vi "process.vi"(8 "error in":errorcluster, 9 "result allocation":T1, 10 "parameters":T1, 11 "module in":refnum<class "tag select module runtime.lvclass">) -> (0 "error out":errorcluster, 1 "results":T1, 2 "parameter allocation":T1, 3 "module out":refnum<class "tag select module runtime.lvclass">)   [LabVIEW 2015, in "tag select module runtime.lvclass"]
doc: "Provides an interface for information processing by a module at runtime. While this interface performs no operations, a child should provide an override which may process data in any manner necessary."
uses:
  tag select module runtime.lvclass
  <vilib>/NI/Tag Bus/table/data table.ctl
  tag select module runtime.lvclass/tag select module runtime.ctl
  <vilib>/NI/Tag Bus/table/data polymorphs/read one/read Boolean.vi
  <vilib>/NI/Tag Bus/table/data polymorphs/read one/read Double.vi
  <vilib>/NI/Tag Bus/table/data polymorphs/write one/write Double.vi
  <vilib>/NI/Tag Bus/table/data polymorphs/read one/read Single.vi
  <vilib>/NI/Tag Bus/table/data polymorphs/write one/write Single.vi
  <vilib>/NI/Tag Bus/table/data polymorphs/read one/read I64.vi
  <vilib>/NI/Tag Bus/table/data polymorphs/write one/write I64.vi
  <vilib>/NI/Tag Bus/table/data polymorphs/read one/read I32.vi
  <vilib>/NI/Tag Bus/table/data polymorphs/write one/write I32.vi
  <vilib>/NI/Tag Bus/table/data polymorphs/read one/read I16.vi
  <vilib>/NI/Tag Bus/table/data polymorphs/write one/write I16.vi
  <vilib>/NI/Tag Bus/table/data polymorphs/read one/read I8.vi
  <vilib>/NI/Tag Bus/table/data polymorphs/write one/write I8.vi
  <vilib>/NI/Tag Bus/table/data polymorphs/read one/read U64.vi
  <vilib>/NI/Tag Bus/table/data polymorphs/write one/write U64.vi
  <vilib>/NI/Tag Bus/table/data polymorphs/read one/read U32.vi
  <vilib>/NI/Tag Bus/table/data polymorphs/write one/write U32.vi
  <vilib>/NI/Tag Bus/table/data polymorphs/read one/read U16.vi
  <vilib>/NI/Tag Bus/table/data polymorphs/write one/write U16.vi
  <vilib>/NI/Tag Bus/table/data polymorphs/read one/read U8.vi
  <vilib>/NI/Tag Bus/table/data polymorphs/write one/write U8.vi
  <vilib>/NI/Tag Bus/table/data polymorphs/write one/write Boolean.vi
  <vilib>/NI/Tag Bus/table/data polymorphs/read one/read String.vi
  <vilib>/NI/Tag Bus/table/data polymorphs/write one/write String.vi
  <vilib>/NI/Tag Bus/table/data polymorphs/read one/read Array of Double.vi
  <vilib>/NI/Tag Bus/table/data polymorphs/write one/write Array of Double.vi
  <vilib>/NI/Tag Bus/table/data polymorphs/read one/read Array of Single.vi
  <vilib>/NI/Tag Bus/table/data polymorphs/write one/write Array of Single.vi
  <vilib>/NI/Tag Bus/table/data polymorphs/read one/read Array of I64.vi
  <vilib>/NI/Tag Bus/table/data polymorphs/write one/write Array of I64.vi
  <vilib>/NI/Tag Bus/table/data polymorphs/read one/read Array of I32.vi
  <vilib>/NI/Tag Bus/table/data polymorphs/write one/write Array of I32.vi
  <vilib>/NI/Tag Bus/table/data polymorphs/read one/read Array of I16.vi
  <vilib>/NI/Tag Bus/table/data polymorphs/write one/write Array of I16.vi
  <vilib>/NI/Tag Bus/table/data polymorphs/read one/read Array of I8.vi
  <vilib>/NI/Tag Bus/table/data polymorphs/write one/write Array of I8.vi
  <vilib>/NI/Tag Bus/table/data polymorphs/read one/read Array of U64.vi
  <vilib>/NI/Tag Bus/table/data polymorphs/write one/write Array of U64.vi
  <vilib>/NI/Tag Bus/table/data polymorphs/read one/read Array of U32.vi
  <vilib>/NI/Tag Bus/table/data polymorphs/write one/write Array of U32.vi
  <vilib>/NI/Tag Bus/table/data polymorphs/read one/read Array of U16.vi
  <vilib>/NI/Tag Bus/table/data polymorphs/write one/write Array of U16.vi
  <vilib>/NI/Tag Bus/table/data polymorphs/read one/read Array of U8.vi
  <vilib>/NI/Tag Bus/table/data polymorphs/write one/write Array of U8.vi
  <vilib>/NI/Tag Bus/table/data polymorphs/read one/read Array of Boolean.vi
  <vilib>/NI/Tag Bus/table/data polymorphs/write one/write Array of Boolean.vi
  <vilib>/NI/Tag Bus/table/data polymorphs/read one/read Array of String.vi
  <vilib>/NI/Tag Bus/table/data polymorphs/write one/write Array of String.vi
  <vilib>/NI/Tag Bus/table/data table.lvlib
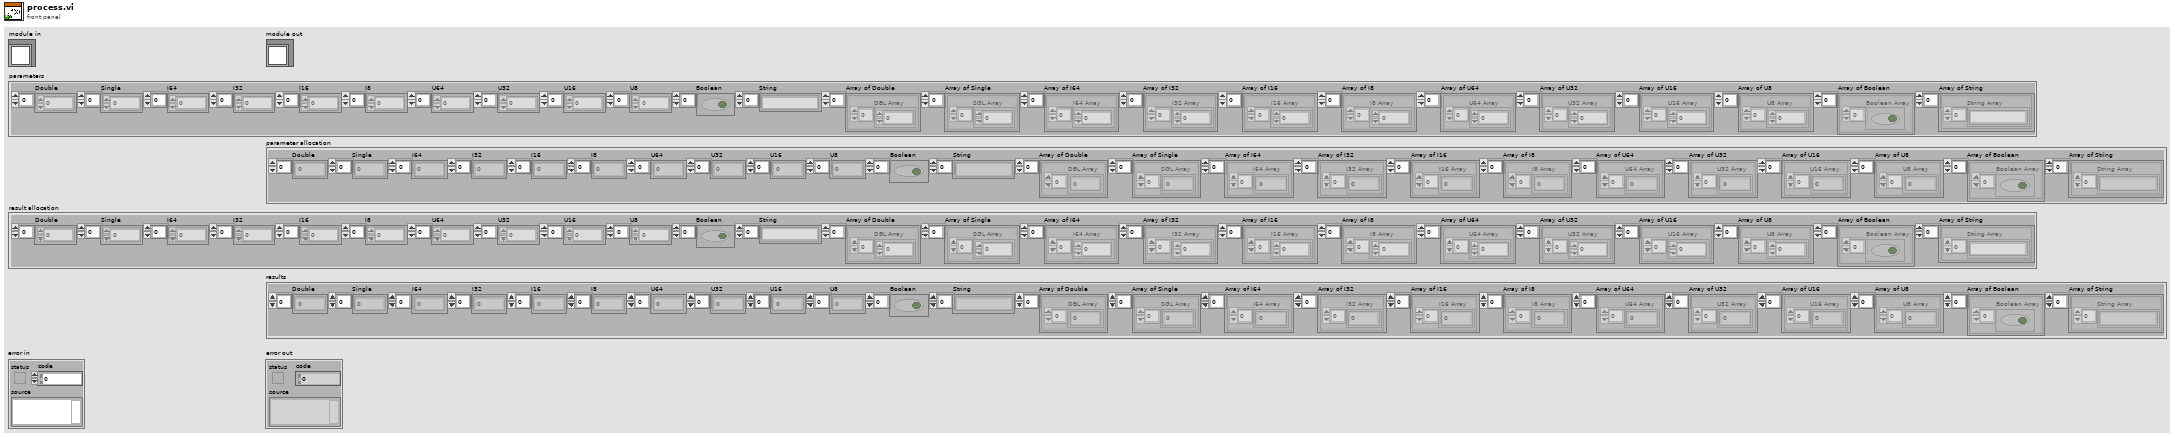
[diagram p1: front panel]
types:
  T1 = typedef "tag bus.lvlib/data table.lvlib/data table.ctl" = cluster{"Double":dbl[], "Single":sgl[], "I64":i64[], "I32":i32[], "I16":i16[], "I8":i8[], "U64":u64[], "U32":u32[], "U16":u16[], "U8":u8[], "Boolean":bool[], "String":string[], "Array of Double":cluster{"DBL Array":dbl[]}[], "Array of Single":cluster{"SGL Array":sgl[]}[], "Array of I64":cluster{"I64 Array":i64[]}[], "Array of I32":cluster{"I32 Array":i32[]}[], "Array of I16":cluster{"I16 Array":i16[]}[], "Array of I8":cluster{"I8 Array":i8[]}[], "Array of U64":cluster{"U64 Array":u64[]}[], "Array of U32":cluster{"U32 Array":u32[]}[], "Array of U16":cluster{"U16 Array":u16[]}[], "Array of U8":cluster{"U8 Array":u8[]}[], "Array of Boolean":cluster{"Boolean Array":bool[]}[], "Array of String":cluster{"String Array":string[]}[]}
  T2 = typedef "tag select module runtime.lvclass/runtime tag select configuration.ctl" = cluster{"output index":i32, "select index (bool)":i32, "input index":i32[], "data type":T3}
  T3 = typedef "tag bus.lvlib/tag descriptor.lvclass/Data Type.ctl" = enum16{"Double", "Single", "I64", "I32", "I16", "I8", "U64", "U32", "U16", "U8", "Boolean", "String", "Array of Double", "Array of Single", "Array of I64", "Array of I32", "Array of I16", "Array of I8", "Array of U64", "Array of U32", "Array of U16", "Array of U8", "Array of Boolean", "Array of String"}
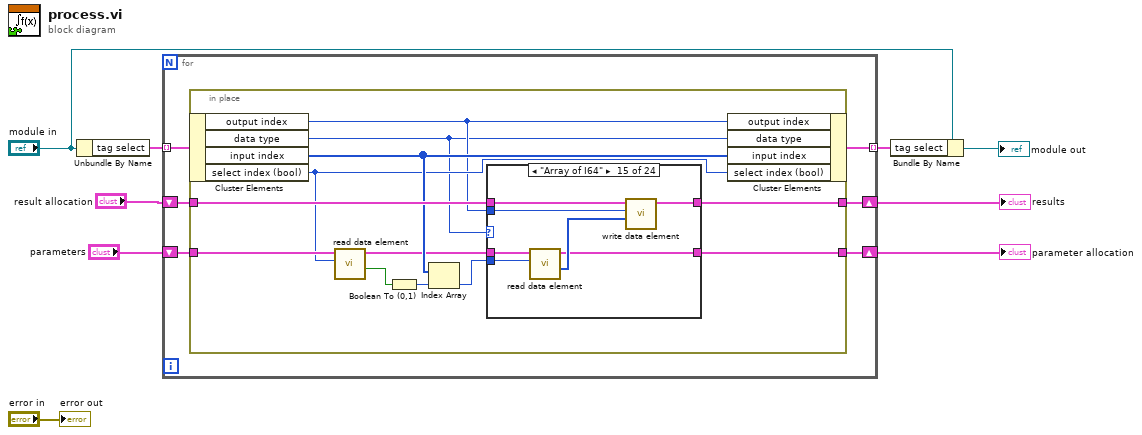
[diagram p0: block diagram]
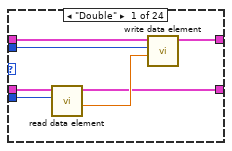
[diagram p2: hidden frame]
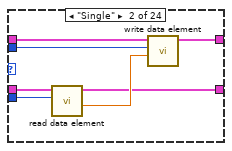
[diagram p3: hidden frame]
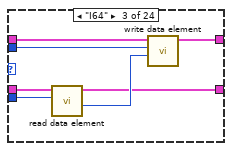
[diagram p4: hidden frame]
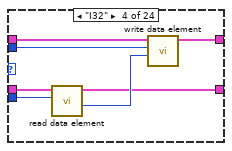
[diagram p5: hidden frame]
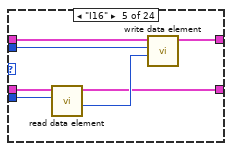
[diagram p6: hidden frame]
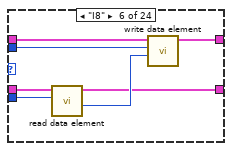
[diagram p7: hidden frame]
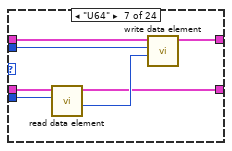
[diagram p8: hidden frame]
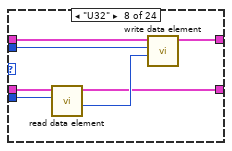
[diagram p9: hidden frame]
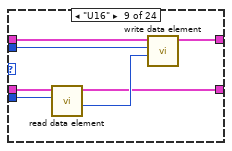
[diagram p10: hidden frame]
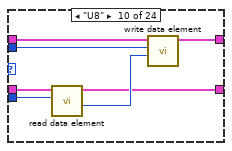
[diagram p11: hidden frame]
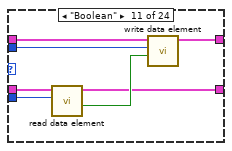
[diagram p12: hidden frame]
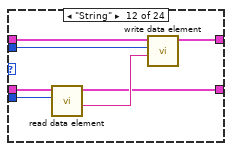
[diagram p13: hidden frame]
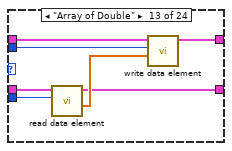
[diagram p14: hidden frame]
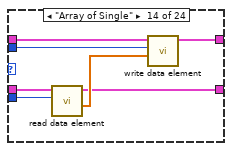
[diagram p15: hidden frame]
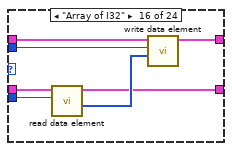
[diagram p16: hidden frame]
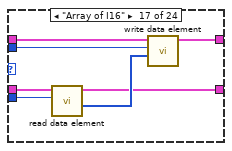
[diagram p17: hidden frame]
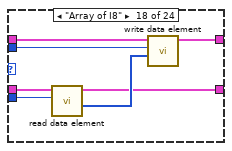
[diagram p18: hidden frame]
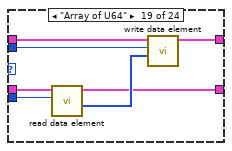
[diagram p19: hidden frame]
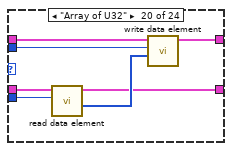
[diagram p20: hidden frame]
diagram:
  n1 = Unbundle By Name("module in") -> ("tag select"=w7:T2[])
  n2 = for {
    tunnel: w7 -> [w15] mode=indexing
    tunnel: [w14] -> w6 mode=indexing
    shift-right: [w10] -> w4
    shift-left: "parameters" -> [w13]
    shift-right: [w11] -> w2
    shift-left: "result allocation" -> [w12]
    n3 = in-place {
      in-place-border: w13 -> [w27]
      in-place-border: w12 -> [w26]
      in-place-border: [w25] -> w11
      in-place-border: [w18] -> w10
      n4 = in-place-cluster #1(w15) -> ("output index"=w17:i32, "data type"=w16:T3, "input index"=w21:i32[], "select index (bool)"=w20:i32)
      n5 = call-poly <vilib>:"read data element.vi"("index"=w20, "data table in"=w27) -> ("value"=w23:bool, "data table out"=w19:T1)  [unwired: 8 in]
      n6 = Boolean To (0,1)(Boolean=w23) -> (0, 1=w24:i16)
      n7 = Index Array(array=w21, index=w24) -> (element=w22:i32)
      n8 = case shown="\"Array of I64\"" w16 {
        tunnel: w26 -> [w28 w35 w42 w49 w56 w63 w70 w77 w84 w91 w98 w105 w112 w119 w126 w133 w140 w147 w154 w161 w168 w175 w182 w189]
        tunnel: [w34 w41 w48 w55 w62 w69 w76 w83 w90 w97 w104 w111 w118 w125 w132 w139 w146 w153 w160 w167 w174 w181 w188 w195] -> w25
        tunnel: w22 -> [w33 w40 w47 w54 w61 w68 w75 w82 w89 w96 w103 w110 w117 w124 w131 w138 w145 w152 w159 w166 w173 w180 w187 w194]
        tunnel: w17 -> [w32 w39 w46 w53 w60 w67 w74 w81 w88 w95 w102 w109 w116 w123 w130 w137 w144 w151 w158 w165 w172 w179 w186 w193]
        tunnel: w19 -> [w30 w37 w44 w51 w58 w65 w72 w79 w86 w93 w100 w107 w114 w121 w128 w135 w142 w149 w156 w163 w170 w177 w184 w191]
        tunnel: [w29 w36 w43 w50 w57 w64 w71 w78 w85 w92 w99 w106 w113 w120 w127 w134 w141 w148 w155 w162 w169 w176 w183 w190] -> w18
        frame "Double" {
          n9 = call-poly <vilib>:"read data element.vi"("index"=w33, "data table in"=w30) -> ("value"=w31:dbl, "data table out"=w29:T1)  [unwired: 8 in]
          n10 = call-poly <vilib>:"write data element.vi"("value"=w31, "index"=w32, "data table in"=w28) -> ("data table out"=w34:T1)  [unwired: 8 in]
        }
        frame "Single" {
          n11 = call-poly <vilib>:"read data element.vi"("index"=w40, "data table in"=w37) -> ("value"=w38:sgl, "data table out"=w36:T1)  [unwired: 8 in]
          n12 = call-poly <vilib>:"write data element.vi"("value"=w38, "index"=w39, "data table in"=w35) -> ("data table out"=w41:T1)  [unwired: 8 in]
        }
        frame "I64" {
          n13 = call-poly <vilib>:"read data element.vi"("index"=w47, "data table in"=w44) -> ("value"=w45:i64, "data table out"=w43:T1)  [unwired: 8 in]
          n14 = call-poly <vilib>:"write data element.vi"("value"=w45, "index"=w46, "data table in"=w42) -> ("data table out"=w48:T1)  [unwired: 8 in]
        }
        frame "I32" {
          n15 = call-poly <vilib>:"read data element.vi"("index"=w54, "data table in"=w51) -> ("value"=w52:i32, "data table out"=w50:T1)  [unwired: 8 in]
          n16 = call-poly <vilib>:"write data element.vi"("value"=w52, "index"=w53, "data table in"=w49) -> ("data table out"=w55:T1)  [unwired: 8 in]
        }
        frame "I16" {
          n17 = call-poly <vilib>:"read data element.vi"("index"=w61, "data table in"=w58) -> ("value"=w59:i16, "data table out"=w57:T1)  [unwired: 8 in]
          n18 = call-poly <vilib>:"write data element.vi"("value"=w59, "index"=w60, "data table in"=w56) -> ("data table out"=w62:T1)  [unwired: 8 in]
        }
        frame "I8" {
          n19 = call-poly <vilib>:"read data element.vi"("index"=w68, "data table in"=w65) -> ("value"=w66:i8, "data table out"=w64:T1)  [unwired: 8 in]
          n20 = call-poly <vilib>:"write data element.vi"("value"=w66, "index"=w67, "data table in"=w63) -> ("data table out"=w69:T1)  [unwired: 8 in]
        }
        frame "U64" {
          n21 = call-poly <vilib>:"read data element.vi"("index"=w75, "data table in"=w72) -> ("value"=w73:u64, "data table out"=w71:T1)  [unwired: 8 in]
          n22 = call-poly <vilib>:"write data element.vi"("value"=w73, "index"=w74, "data table in"=w70) -> ("data table out"=w76:T1)  [unwired: 8 in]
        }
        frame "U32" {
          n23 = call-poly <vilib>:"read data element.vi"("index"=w82, "data table in"=w79) -> ("value"=w80:u32, "data table out"=w78:T1)  [unwired: 8 in]
          n24 = call-poly <vilib>:"write data element.vi"("value"=w80, "index"=w81, "data table in"=w77) -> ("data table out"=w83:T1)  [unwired: 8 in]
        }
        frame "U16" {
          n25 = call-poly <vilib>:"read data element.vi"("index"=w89, "data table in"=w86) -> ("value"=w87:u16, "data table out"=w85:T1)  [unwired: 8 in]
          n26 = call-poly <vilib>:"write data element.vi"("value"=w87, "index"=w88, "data table in"=w84) -> ("data table out"=w90:T1)  [unwired: 8 in]
        }
        frame "U8" {
          n27 = call-poly <vilib>:"read data element.vi"("index"=w96, "data table in"=w93) -> ("value"=w94:u8, "data table out"=w92:T1)  [unwired: 8 in]
          n28 = call-poly <vilib>:"write data element.vi"("value"=w94, "index"=w95, "data table in"=w91) -> ("data table out"=w97:T1)  [unwired: 8 in]
        }
        frame "Boolean" {
          n29 = call-poly <vilib>:"read data element.vi"("index"=w103, "data table in"=w100) -> ("value"=w101:bool, "data table out"=w99:T1)  [unwired: 8 in]
          n30 = call-poly <vilib>:"write data element.vi"("value"=w101, "index"=w102, "data table in"=w98) -> ("data table out"=w104:T1)  [unwired: 8 in]
        }
        frame "String" {
          n31 = call-poly <vilib>:"read data element.vi"("index"=w110, "data table in"=w107) -> ("value"=w108:string, "data table out"=w106:T1)  [unwired: 8 in]
          n32 = call-poly <vilib>:"write data element.vi"("value"=w108, "index"=w109, "data table in"=w105) -> ("data table out"=w111:T1)  [unwired: 8 in]
        }
        frame "Array of Double" {
          n33 = call-poly <vilib>:"read data element.vi"("index"=w117, "data table in"=w114) -> ("value"=w115:dbl[], "data table out"=w113:T1)  [unwired: 8 in]
          n34 = call-poly <vilib>:"write data element.vi"("value"=w115, "index"=w116, "data table in"=w112) -> ("data table out"=w118:T1)  [unwired: 8 in]
        }
        frame "Array of Single" {
          n35 = call-poly <vilib>:"read data element.vi"("index"=w124, "data table in"=w121) -> ("value"=w122:sgl[], "data table out"=w120:T1)  [unwired: 8 in]
          n36 = call-poly <vilib>:"write data element.vi"("value"=w122, "index"=w123, "data table in"=w119) -> ("data table out"=w125:T1)  [unwired: 8 in]
        }
        frame "Array of I64" {
          n37 = call-poly <vilib>:"read data element.vi"("index"=w131, "data table in"=w128) -> ("value"=w129:i64[], "data table out"=w127:T1)  [unwired: 8 in]
          n38 = call-poly <vilib>:"write data element.vi"("value"=w129, "index"=w130, "data table in"=w126) -> ("data table out"=w132:T1)  [unwired: 8 in]
        }
        frame "Array of I32" {
          n39 = call-poly <vilib>:"read data element.vi"("index"=w138, "data table in"=w135) -> ("value"=w136:i32[], "data table out"=w134:T1)  [unwired: 8 in]
          n40 = call-poly <vilib>:"write data element.vi"("value"=w136, "index"=w137, "data table in"=w133) -> ("data table out"=w139:T1)  [unwired: 8 in]
        }
        frame "Array of I16" {
          n41 = call-poly <vilib>:"read data element.vi"("index"=w145, "data table in"=w142) -> ("value"=w143:i16[], "data table out"=w141:T1)  [unwired: 8 in]
          n42 = call-poly <vilib>:"write data element.vi"("value"=w143, "index"=w144, "data table in"=w140) -> ("data table out"=w146:T1)  [unwired: 8 in]
        }
        frame "Array of I8" {
          n43 = call-poly <vilib>:"read data element.vi"("index"=w152, "data table in"=w149) -> ("value"=w150:i8[], "data table out"=w148:T1)  [unwired: 8 in]
          n44 = call-poly <vilib>:"write data element.vi"("value"=w150, "index"=w151, "data table in"=w147) -> ("data table out"=w153:T1)  [unwired: 8 in]
        }
        frame "Array of U64" {
          n45 = call-poly <vilib>:"read data element.vi"("index"=w159, "data table in"=w156) -> ("value"=w157:u64[], "data table out"=w155:T1)  [unwired: 8 in]
          n46 = call-poly <vilib>:"write data element.vi"("value"=w157, "index"=w158, "data table in"=w154) -> ("data table out"=w160:T1)  [unwired: 8 in]
        }
        frame "Array of U32" {
          n47 = call-poly <vilib>:"read data element.vi"("index"=w166, "data table in"=w163) -> ("value"=w164:u32[], "data table out"=w162:T1)  [unwired: 8 in]
          n48 = call-poly <vilib>:"write data element.vi"("value"=w164, "index"=w165, "data table in"=w161) -> ("data table out"=w167:T1)  [unwired: 8 in]
        }
        frame "Array of U16" {
          n49 = call-poly <vilib>:"read data element.vi"("index"=w173, "data table in"=w170) -> ("value"=w171:u16[], "data table out"=w169:T1)  [unwired: 8 in]
          n50 = call-poly <vilib>:"write data element.vi"("value"=w171, "index"=w172, "data table in"=w168) -> ("data table out"=w174:T1)  [unwired: 8 in]
        }
        frame "Array of U8" {
          n51 = call-poly <vilib>:"read data element.vi"("index"=w180, "data table in"=w177) -> ("value"=w178:u8[], "data table out"=w176:T1)  [unwired: 8 in]
          n52 = call-poly <vilib>:"write data element.vi"("value"=w178, "index"=w179, "data table in"=w175) -> ("data table out"=w181:T1)  [unwired: 8 in]
        }
        frame "Array of Boolean" {
          n53 = call-poly <vilib>:"read data element.vi"("index"=w187, "data table in"=w184) -> ("value"=w185:bool[], "data table out"=w183:T1)  [unwired: 8 in]
          n54 = call-poly <vilib>:"write data element.vi"("value"=w185, "index"=w186, "data table in"=w182) -> ("data table out"=w188:T1)  [unwired: 8 in]
        }
        frame "Array of String" {
          n55 = call-poly <vilib>:"read data element.vi"("index"=w194, "data table in"=w191) -> ("value"=w192:string[], "data table out"=w190:T1)  [unwired: 8 in]
          n56 = call-poly <vilib>:"write data element.vi"("value"=w192, "index"=w193, "data table in"=w189) -> ("data table out"=w195:T1)  [unwired: 8 in]
        }
      }
      n57 = in-place-cluster #1("output index"=w17, "data type"=w16, "input index"=w21, "select index (bool)"=w20) -> (w14:T2)
    }
  }
  "results" <- w2
  "parameter allocation" <- w4
  n58 = Bundle By Name(cluster="module in", "tag select"=w6) -> (→"module out":refnum<class "tag select module runtime.lvclass">)
  "error out" <- "error in"
